vi "Test_Manual_BP4610.vi"() -> ()   [LabVIEW 2019]
uses:
  Type def/SetNF_BP4610.ctl
  Type def/limitNF_4610.ctl
panel:
  in  "Limit":bool
  in  "LimitBP":T1={"Set"=enum."Current", "Voltage+[V]"=20.0, "Current+[A]"=5.0, "Voltage-[V]"=-20.0, "Current-[A]"=-5.0} {"Current-[A]" min=-20.0 max=20.0 step=0.001; "Voltage-[V]" min=-115.0 max=115.0 step=0.01; "Current+[A]" min=0.0 max=60.0 step=0.01; "Voltage+[V]" min=0.0 max=120.0 step=0.1}
  in  "Set BP":T2={"Set"=enum."FREQ/WAVE", "Operation mode"=0, "Voltage[Vp-p]"=0.0, "Current[Ap-p]"=0.0, "Voltage[V]"=0.0, "Current[A]"=0.0, "Frequency[Hz]"=1.0, "Waveform"=enum."Sine"} {"Frequency[Hz]" min=1.0 max=100000.0 step=0.1; "Current[A]" min=-20.0 max=20.0 step=0.001; "Voltage[V]" min=-115.0 max=115.0 step=0.01; "Current[Ap-p]" min=0.0 max=60.0 step=0.01; "Voltage[Vp-p]" min=0.0 max=120.0 step=0.1; "Operation mode" items=["CV-INT", "CV-EXT", "CV-ADD", "CC-INT", "CC-EXT", "CC-ADD"]}
  in  "Set":bool
  in  "port":refnum<visa-resource-name> caption="VISAsession"
  in  "read":bool
  in  "output":bool
  out "DC current[A]":dbl format="%.2f"
  out "DC voltage[V]":dbl format="%.1f"
  in  "stop":bool
  in  "close":bool
  in  "open":bool
  # "NF BP4610"
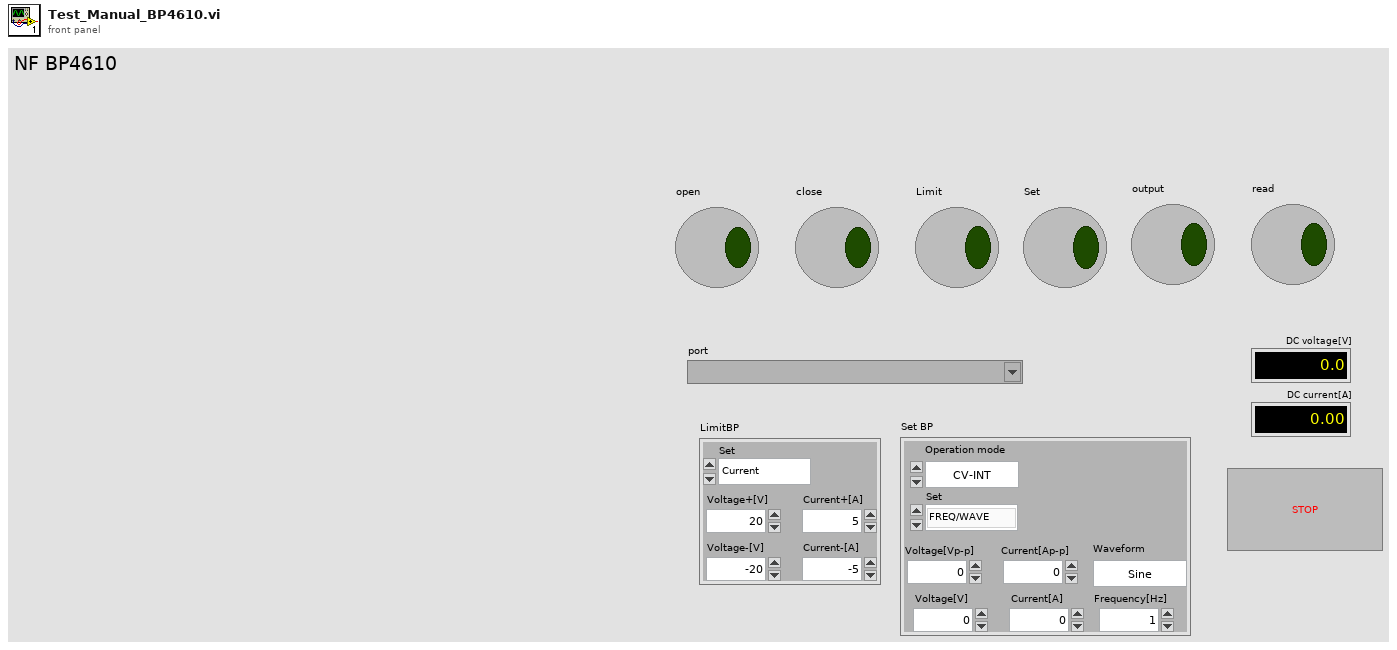
[diagram p1: front panel]
types:
  T1 = typedef "limitNF_4610.ctl" = cluster{"Set":enum16{"Current", "Voltage"}, "Voltage+[V]":dbl, "Current+[A]":dbl, "Voltage-[V]":dbl, "Current-[A]":dbl}
  T2 = typedef "SetNF_BP4610.ctl" = cluster{"Set":enum16{"Current", "Voltage", "FREQ/WAVE"}, "Operation mode":u16, "Voltage[Vp-p]":dbl, "Current[Ap-p]":dbl, "Voltage[V]":dbl, "Current[A]":dbl, "Frequency[Hz]":dbl, "Waveform":enum16{"Sine", "Square", "ARB 1", "ARB 2", "ARB 3", "ARB 4", "ARB 5", "ARB 6", "ARB 7", "ARB 8", "ARB 9", "ARB 10", "ARB 11", "ARB 12", "ARB 13", "ARB 14", "ARB 15", "ARB 16"}}
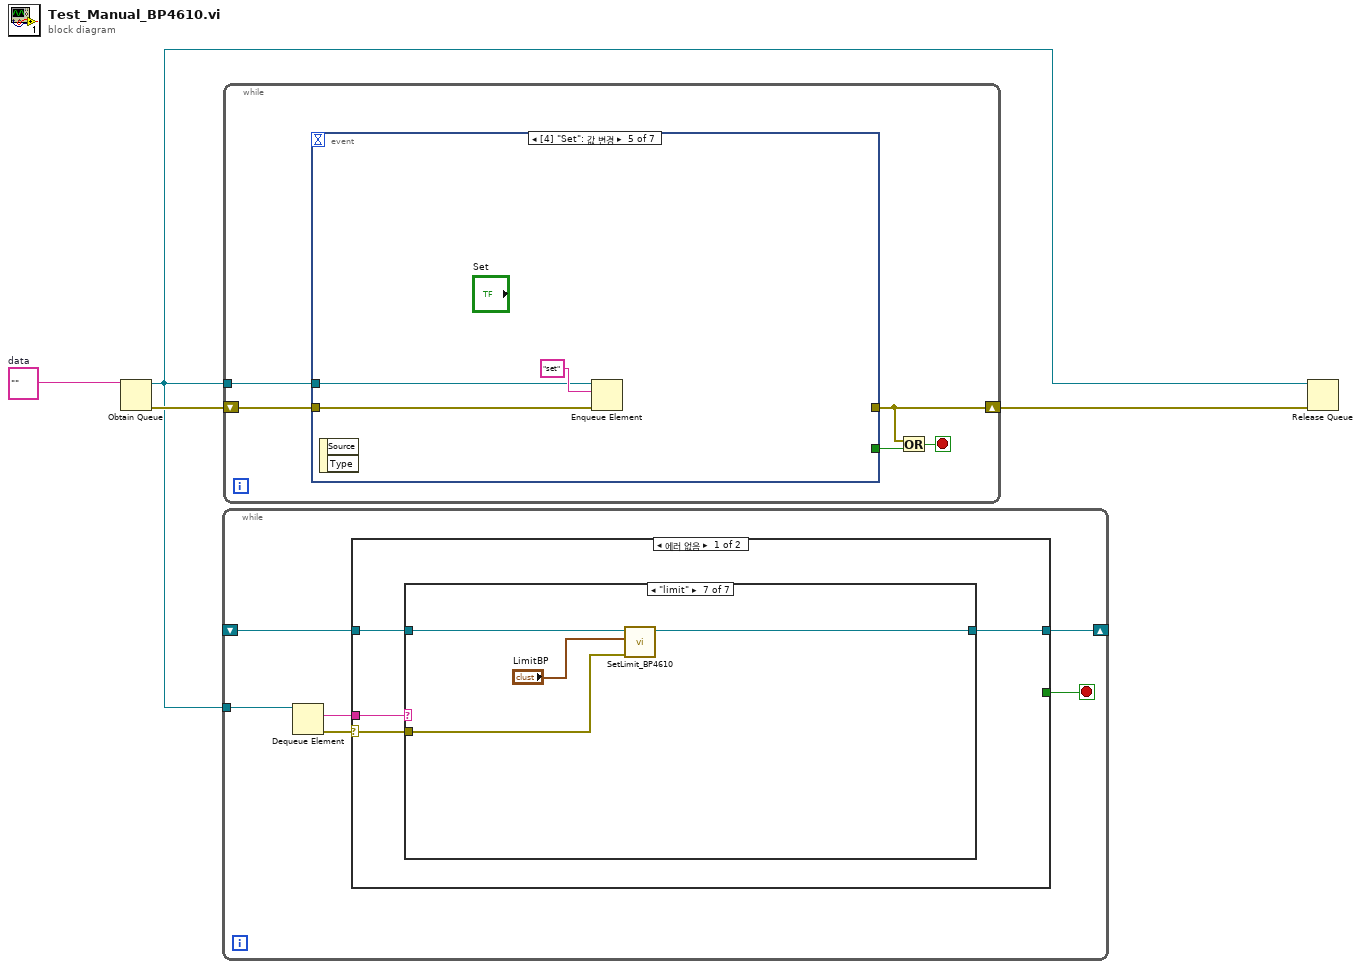
[diagram p0: block diagram]
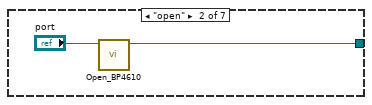
[diagram p3: hidden frame]
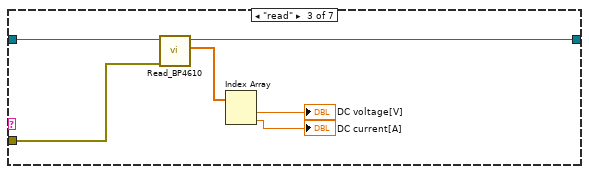
[diagram p4: hidden frame]
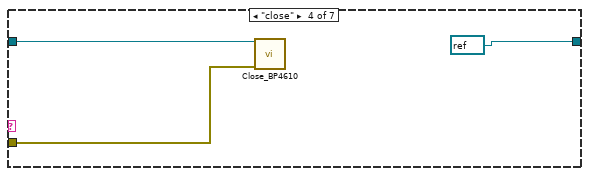
[diagram p5: hidden frame]
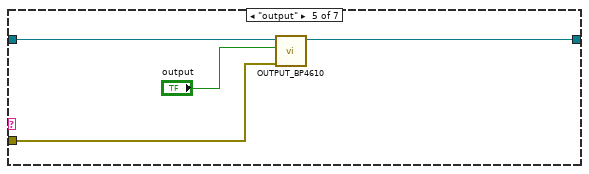
[diagram p6: hidden frame]
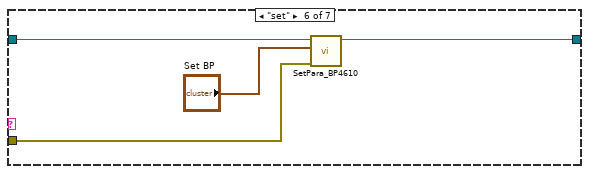
[diagram p7: hidden frame]
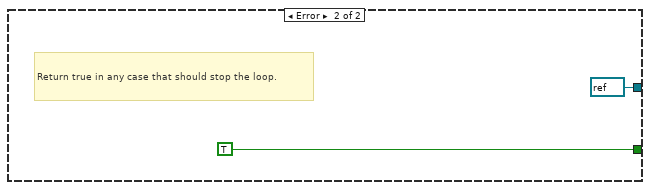
[diagram p8: hidden frame]
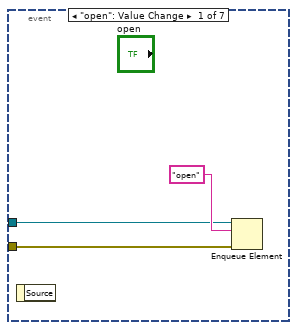
[diagram p9: hidden frame]
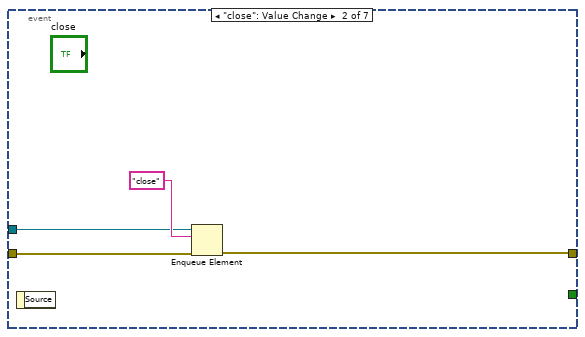
[diagram p10: hidden frame]
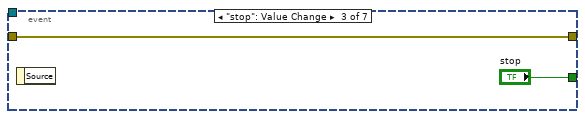
[diagram p11: hidden frame]
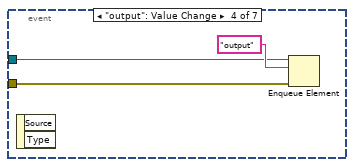
[diagram p12: hidden frame]
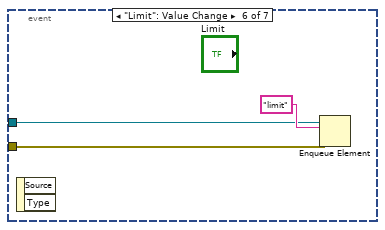
[diagram p13: hidden frame]
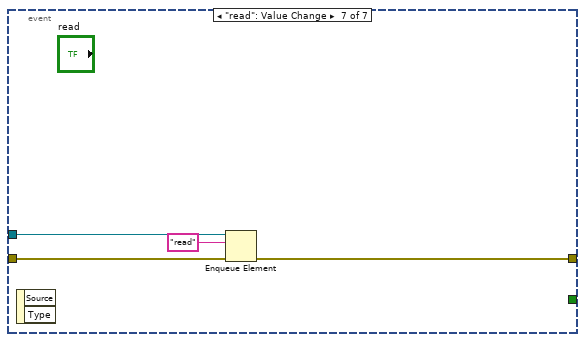
[diagram p14: hidden frame]
diagram:
  w2 = ""  # data
  n1 = Obtain Queue(element data type=w2) -> (queue out=w1:refnum<queue>, error out=w4:errorcluster)  [unwired: 4 in, 1 out]
  n2 = while {
    tunnel: w1 -> [w10]
    shift-right: [w6] -> _
    shift-left: _ -> [w5]
    stop <- w7 stop-if-true
    n3 = Dequeue Element(queue=w10) -> (element=w8:string, error out=w9:errorcluster)  [unwired: 2 in, 2 out]
    n4 = case shown="에러 없음" w9 {
      selector: w9 -> [w11 _]
      tunnel: w8 -> [w14 _]
      tunnel: [_ TRUE] -> w7
      tunnel: [w13 refnum<visa-resource-name> refnum ("CopyVISAsession")] -> w6
      tunnel: w5 -> [w12 _]
      frame No Error {
        n5 = case shown="\"limit\"" w14 {
          tunnel: [w15 w16 w22 refnum<visa-resource-name> refnum ("CopyVISAsession") w29 w33 w37] -> w13
          tunnel: w12 -> [w15 _ w23 w26 w30 w34 w38]
          tunnel: w11 -> [_ _ w21 w25 w28 w31 w36]
          frame "False", Default {
          }
          frame "open" {
            n6 = call "Open_BP4610.vi"("VISAsession"="port") -> ("CopyVISAsession"=w16:refnum<visa-resource-name>)  [unwired: 9 in, 1 out]
          }
          frame "read" {
            n7 = call "Read_BP4610.vi"("error in (no error)"=w21, "VISAsession"=w23) -> ("Data"=w20:dbl[], "CopyVISAsession"=w22:refnum<visa-resource-name>)  [unwired: 7 in, 1 out]
            n8 = Index Array(array=w20) -> (element #1=→"DC voltage[V]":dbl, element #2=→"DC current[A]":dbl)  [unwired: 2 in]
          }
          frame "close" {
            n9 = call "Close_BP4610.vi"("error in"=w25, "VISA"=w26) -> ()  [unwired: 9 in, 1 out]
          }
          frame "output" {
            n10 = call "OUTPUT_BP4610.vi"("error in"=w28, "Output"="output", "port in"=w30) -> ("port out"=w29:refnum<visa-resource-name>)  [unwired: 7 in, 1 out]
          }
          frame "set" {
            n11 = call "SetPara_BP4610.vi"("error in"=w31, "SetBP"="Set BP", "VISA"=w34) -> ("VISA out"=w33:refnum<visa-resource-name>)  [unwired: 7 in, 1 out]
          }
          frame "limit" {
            n12 = call "SetLimit_BP4610.vi"("error in"=w36, "LimitBP"="LimitBP", "VISA"=w38) -> ("VISA out"=w37:refnum<visa-resource-name>)  [unwired: 7 in, 1 out]
          }
        }
      }
      frame Error {
        # "Return true in any case that should stop the loop."
      }
    }
  }
  n13 = while {
    shift-right: [w41] -> w3
    shift-left: w4 -> [w44]
    tunnel: w1 -> [w45]
    stop <- w42 stop-if-true
    n14 = event shown="[4] \"Set\": 값 변경" {
      selector: _ -> [_ _ _ _ _ _ _]
      dyn-events: _ -> [_ _ _ _ _ _ _]
      timeout: _ -> [_ _ _ _ _ _ _]
      tunnel: w45 -> [w47 w51 _ w56 w59 w62 w66]
      tunnel: w44 -> [w46 w50 w53 w55 w58 w61 w65]
      tunnel: [_ w49 w53 _ _ _ w64] -> w41
      tunnel: [_ _ "stop" _ _ _ _] -> w43
      event "open": Value Change {
        n15 = event-data() -> ()  [unwired: 1 in, 1 out]
        n16 = Enqueue Element(queue=w47, element="open", error in (no error)=w46) -> ()  [unwired: 1 in, 3 out]
      }
      event "close": Value Change {
        n17 = event-data() -> ()  [unwired: 1 in, 1 out]
        n18 = Enqueue Element(queue=w51, element="close", error in (no error)=w50) -> (error out=w49:errorcluster)  [unwired: 1 in, 2 out]
      }
      event "stop": Value Change {
        n19 = event-data() -> ()  [unwired: 1 in, 1 out]
      }
      event "output": Value Change {
        n20 = event-data() -> ()  [unwired: 1 in, 2 out]
        n21 = Enqueue Element(queue=w56, element="output", error in (no error)=w55) -> ()  [unwired: 1 in, 3 out]
      }
      event "Set": Value Change {
        n22 = event-data() -> ()  [unwired: 1 in, 2 out]
        n23 = Enqueue Element(queue=w59, element="set", error in (no error)=w58) -> ()  [unwired: 1 in, 3 out]
      }
      event "Limit": Value Change {
        n24 = event-data() -> ()  [unwired: 1 in, 2 out]
        n25 = Enqueue Element(queue=w62, element="limit", error in (no error)=w61) -> ()  [unwired: 1 in, 3 out]
      }
      event "read": Value Change {
        n26 = event-data() -> ()  [unwired: 1 in, 2 out]
        n27 = Enqueue Element(queue=w66, element="read", error in (no error)=w65) -> (error out=w64:errorcluster)  [unwired: 1 in, 2 out]
      }
    }
    n28 = Or(x=w41, y=w43) -> (x .or. y?=w42:bool)
  }
  n29 = Release Queue(queue=w1, error in (no error)=w3) -> ()  [unwired: 1 in, 3 out]
